vi "sinewave.vi"() -> ()   [LabVIEW 2023]
panel:
  out "Waveform Chart":dbl(graph)
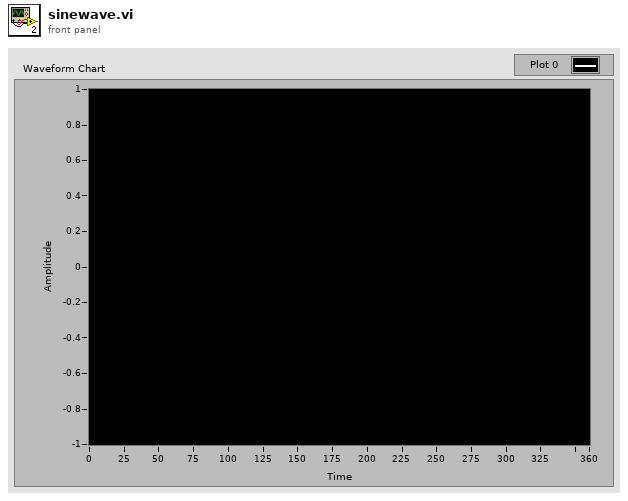
[diagram p1: front panel]
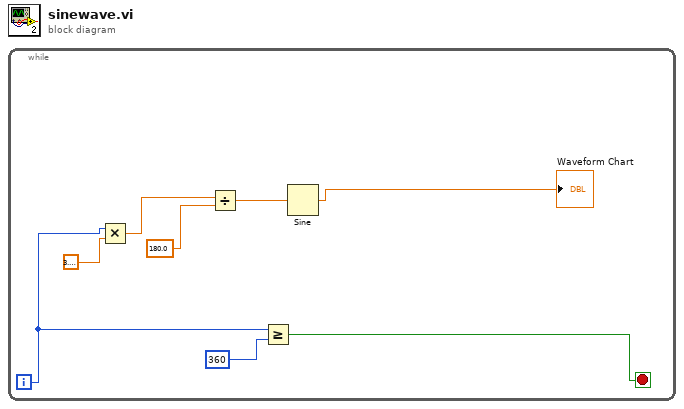
[diagram p0: block diagram]
diagram:
  n1 = while {
    i -> [w4]
    stop <- w6 stop-if-true
    n2 = Multiply(x=w4, y=3.141592653589793) -> (x*y=w5:dbl)
    n3 = Divide(x=w5, y=180.0) -> (x/y=w8:dbl)
    n4 = Greater Or Equal?(x=w4, y=360) -> (x >= y?=w6:bool)
    n5 = Sine(x=w8) -> (sin(x)=→"Waveform Chart":dbl)
  }
